vi "Read Data Package.vi"(8 "Error In":errorcluster, 10 "Data":string, 11 "reference in":refnum<class "CommunicationModule.lvclass">) -> (0 "Error Out":errorcluster, 3 "reference out":refnum<class "CommunicationModule.lvclass">)   [LabVIEW 2024, in "CommunicationModule.lvclass"]
uses:
  CommunicationModule.lvclass
  CommunicationModule.lvclass/CommunicationModule.ctl
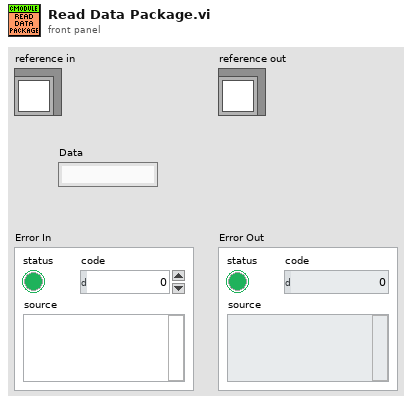
[diagram p1: front panel]
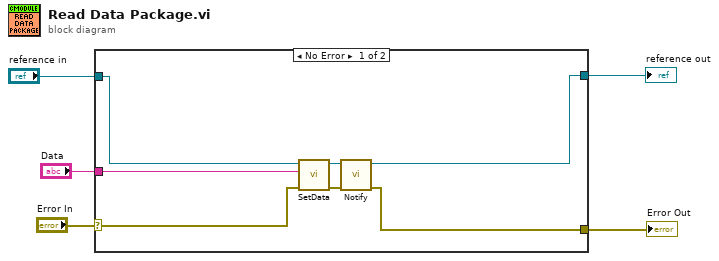
[diagram p0: block diagram]
diagram:
  n1 = case shown="No Error" "Error In" {
    selector: "Error In" -> [w8 w14]
    tunnel: [w10 w14] -> w4
    tunnel: [w11 w13] -> w2
    tunnel: "reference in" -> [w12 w13]
    tunnel: "Data" -> [w7 _]
    frame No Error {
      n2 = call-dynamic "SetData.vi"("Error In"=w8, "Data"=w7, "reference in"=w12) -> ("Error Out"=w6:errorcluster, "reference out"=w9:refnum<class "CommunicationModule.lvclass">)  [unwired: 7 in]
      n3 = call-dynamic "Notify.vi"("Error In"=w6, "reference in"=w9) -> ("Error Out"=w10:errorcluster, "reference out"=w11:refnum<class "CommunicationModule.lvclass">)  [unwired: 8 in]
    }
    frame Error {
    }
  }
  "Error Out" <- w4
  "reference out" <- w2
